vi "Keithley 2002 Disp2 Read.vi"(0 "GPIB address":string="16", 1 "error in":T1) -> (2 "primary display":string, 3 "secondary display":string, 4 "error out":T1)   [LabVIEW 2020]
doc: "This VI is used to read the primary and secondary display of the instrument. The primary display is selected from and of the function config VI's, while the secondary display is selected from the Disp2 Config VI."
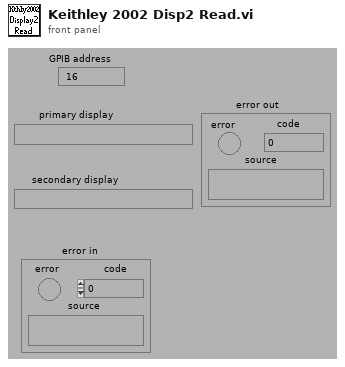
[diagram p1: front panel]
types:
  T1 = cluster{"error":bool, "code":i32, "source":string}
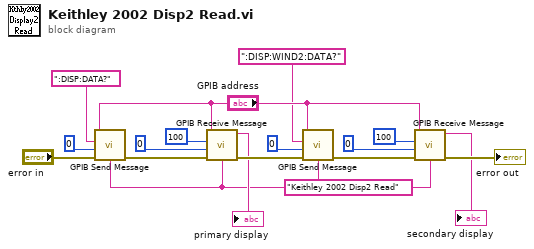
[diagram p0: block diagram]
diagram:
  w1 = "Keithley 2002 Disp2 Read"
  n1 = call "GPIB Send Message.vi"("address string"="GPIB address", "write buffer"=":DISP:DATA?", "source"=w1, "write mode (set END:0)"=0, "error in"="error in") -> ("error out"=w15:T1)  [unwired: 2 in, 2 out]
  n2 = call "GPIB Receive Message.vi"("address string"="GPIB address", "byte count"=100, "source"=w1, "read mode"=0, "error in"=w15) -> ("read buffer"=→"primary display":string, "error out"=w9:T1)  [unwired: 2 in, 1 out]
  n3 = call "GPIB Send Message.vi"("address string"="GPIB address", "write buffer"=":DISP:WIND2:DATA?", "source"=w1, "write mode (set END:0)"=0, "error in"=w9) -> ("error out"=w8:T1)  [unwired: 2 in, 2 out]
  n4 = call "GPIB Receive Message.vi"("address string"="GPIB address", "byte count"=100, "source"=w1, "read mode"=0, "error in"=w8) -> ("read buffer"=→"secondary display":string, "error out"=→"error out":T1)  [unwired: 2 in, 1 out]
